vi "Window-Exporting 8bit videos.vi"(9 "Input cluster":T2) -> ()   [LabVIEW 2013]
uses:
  <vilib>/vision/Avi.llb/IMAQ AVI2 Refnum.ctl
  Patch-Vol video generator/Typedefs/Bright-Contr-Gamma cluster.ctl
  Typedefs/Speed graph behaviour enum.ctl
  Typedefs/8-bit video export window ctrl refs.ctl
  Functional Imaging Viewer/Typedefs/Get-Set-Clear Control.ctl
  Patch-Vol video generator/Globals/gl_8-bit montage window ctrl refs.vi
  Globals/gl_Time series viewer globals.vi
  <vilib>/Utility/miscctls.llb/LVPointTypeDef.ctl
panel:
  out "max value":dbl format="Max intensity value: %#_g"
  out "Progress...":u8(slide) scale=0.0..100.0
  out "Progress indicator":string
  out "Pause":bool
  out "Number of frames":i32 format="Number of frames: %.0f"
  out "split file frame index (0 based)":u32
  out "AVI mode":string
  out "Timelapse frame's global number":i32
  out "8-bit":T3(plugin-control) caption="8-bit video to be exported"
  out "16-bit":T3(plugin-control) caption="Original 16-bit video"
  out "AVI2 split file ref":T1
  in  "Include camera videos":bool
  in  "Include speed graph":bool
  in  "Speed graph behaviour":T4
  in  "Micr. Img Adjstmnt":T5={"Brightness"=1000.0, "Contrast"=45.0, "Gamma"=1.0} {"Gamma" min=0.5 scale=0.0..2.0; "Contrast" min=0.5 scale=0.0..90.0; "Brightness" min=0.5 scale=0.0..30000.0}
  out "Stop (ind)":bool
  out "Exporting":bool
  out "Close":bool
  in  "Stop":bool
  in  "Export":bool
  in  "Play":bool
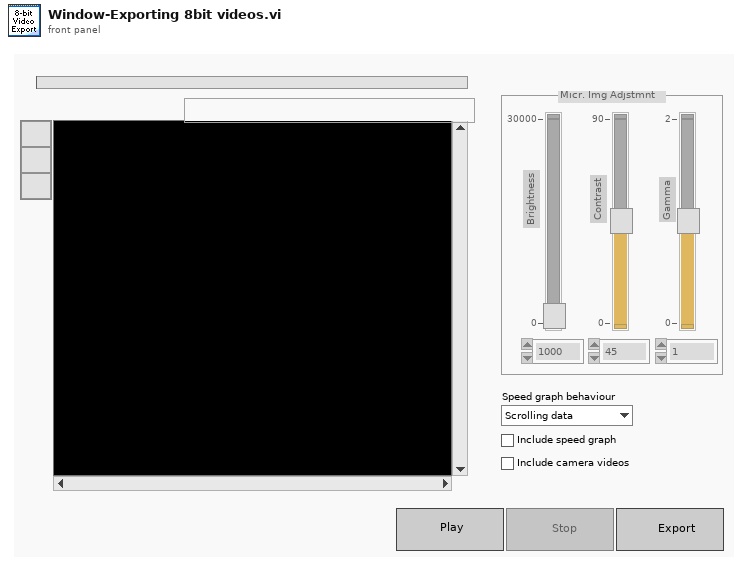
[diagram p1: front panel]
types:
  T1 = typedef "IMAQ AVI2 Refnum.ctl" = refnum<k20>
  T2 = cluster{"# of frames to export":i32, "Initial frame's owning file":T1, "8-bit AVI file path":path, "Cursors location":cluster{"Number of first frame":i32, "Number of last frame":i32}}
  T3 = typedef "IMAQ Image.ctl" = refnum<image>
  T4 = typedef "Speed graph behaviour enum.ctl" = enum16{"Scrolling data", "Scrolling cursor"}
  T5 = typedef "Bright-Contr-Gamma cluster.ctl" = cluster{"Brightness":sgl, "Contrast":sgl, "Gamma":sgl}
  T6 = typedef "8-bit video export window ctrl refs.ctl" = cluster{"Add speed data":refnum<vi>, "Add camera videos":refnum<vi>, "Stop button":refnum<vi>, "Camera Video Adjustments":refnum<vi>, "Microscope Image Adjustments":refnum<vi>, "Execute":refnum<vi>, "Codec":refnum<vi>, "Channel":refnum<vi>, "Speed graph behaviour":refnum<vi>, "Include speed graph":refnum<vi>}
  T7 = cluster{"Number of first frame":i32, "Number of last frame":i32}
  T8 = typedef "LVPointTypeDef.ctl" = cluster{"Horizontal":i16, "Vertical":i16}
  T9 = enum8{"Enabled", "Disabled", "Disabled and Grayed Out"}
  T10 = typedef "Get-Set-Clear Control.ctl" = enum16{"Get", "Set", "Clear"}
  T11 = typedef "Image Type" = u32
  T12 = typedef "AVI modes refs cluster.ctl" = cluster{"AVI1 ref":T13, "AVI2 refs":T1[], "AVI # frames":u32[]}
  T13 = typedef "AviRefnum.ctl" = refnum<k1>
  T14 = enum32{"Invalid", "Standard", "Closed", "Hidden", "Minimized", "Maximized"}
  T15 = typedef "8-bit video export AVI modes cluster.ctl" = cluster{"AVI1 ref":T13, "AVI2 ref":T1, "AVI path":path}
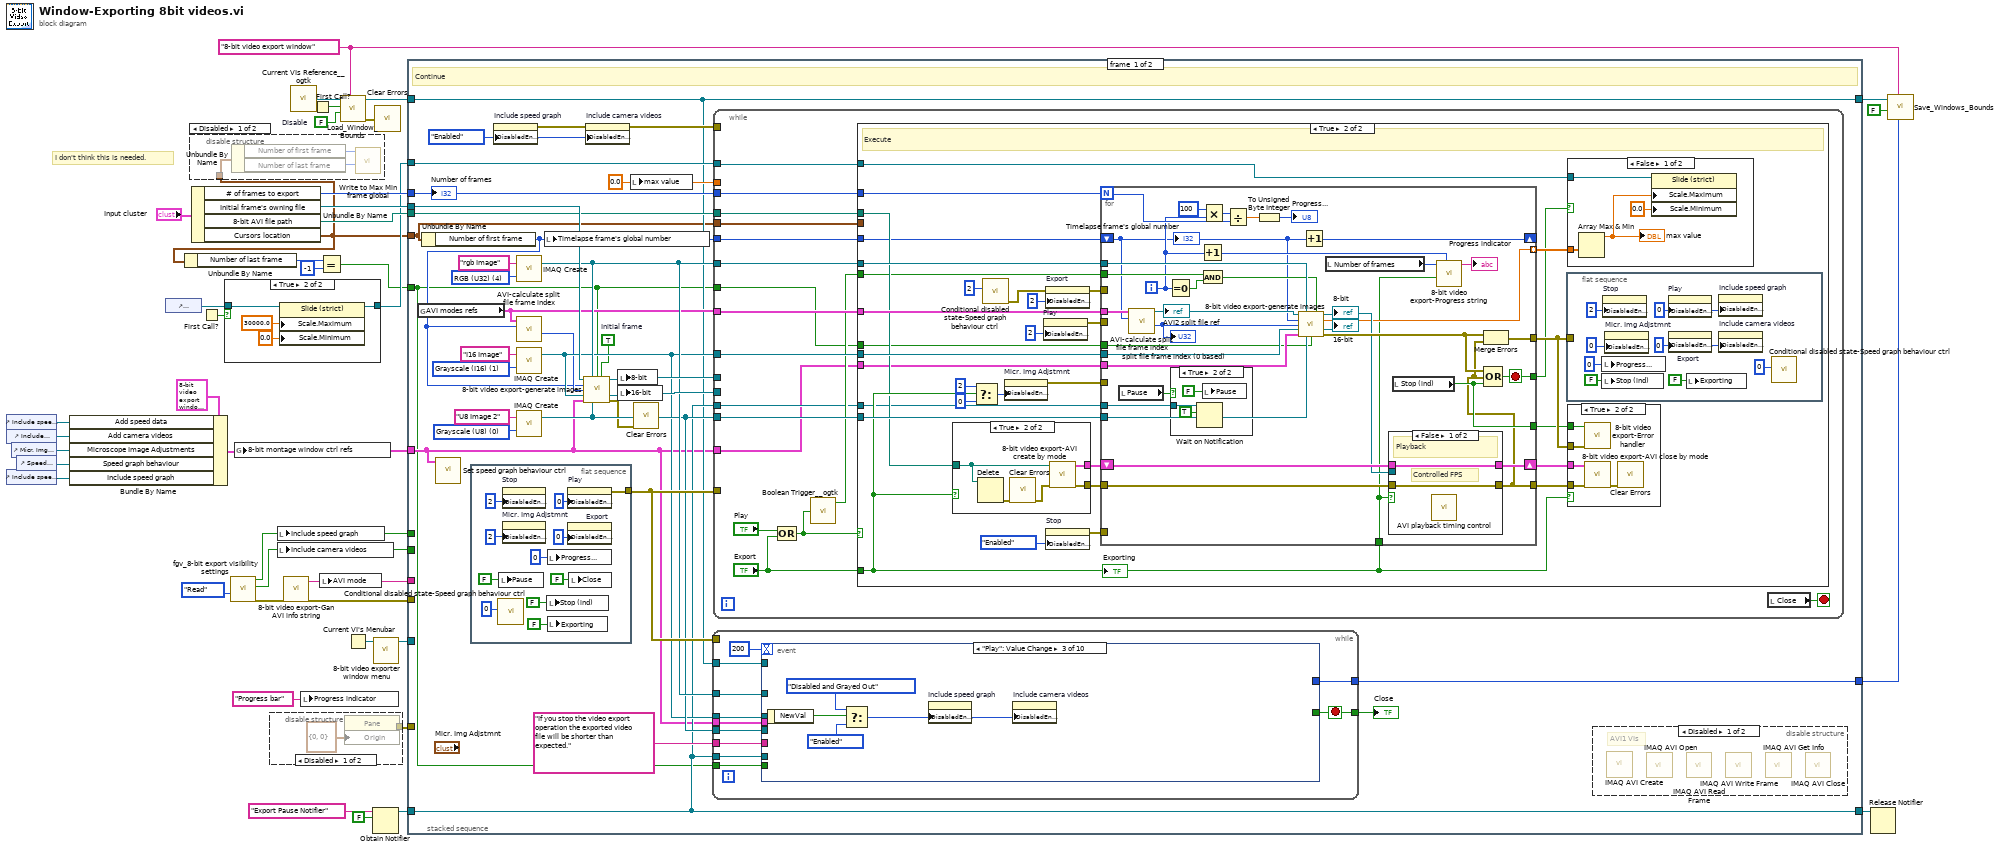
[diagram p0: block diagram]
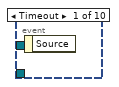
[diagram p6: hidden frame]
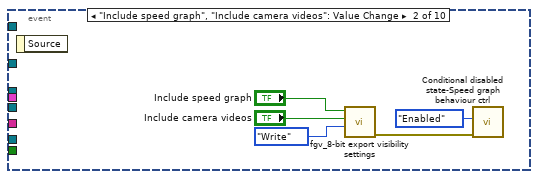
[diagram p7: hidden frame]
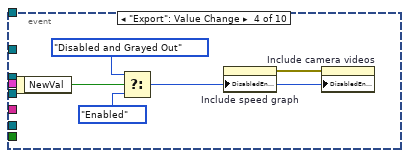
[diagram p8: hidden frame]
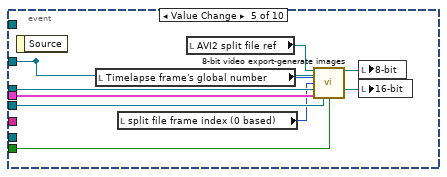
[diagram p9: hidden frame]
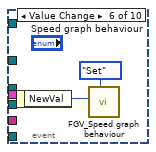
[diagram p10: hidden frame]
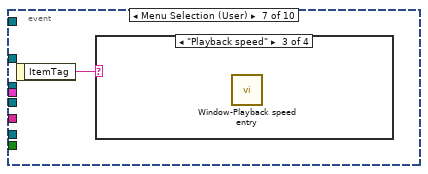
[diagram p11: hidden frame]
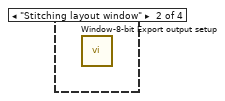
[diagram p13: hidden frame]
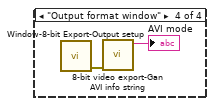
[diagram p14: hidden frame]
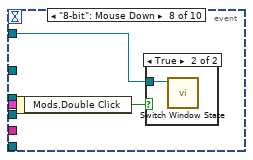
[diagram p15: hidden frame]
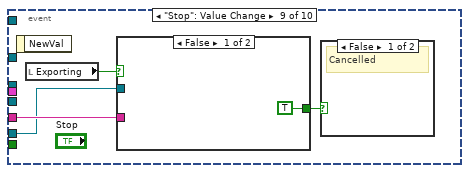
[diagram p17: hidden frame]
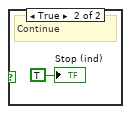
[diagram p18: hidden frame]
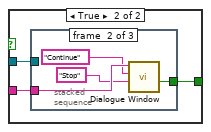
[diagram p19: hidden frame]
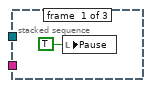
[diagram p20: hidden frame]
diagram:
  w36 = FALSE  # Disable
  w39 = "8-bit video export window" ("Window Name (i.e. Key)")
  # "I don't think this is needed."
  n1 = control-ref of="Include speed graph"() -> (w26:refnum<vi>)
  n2 = control-ref of="Include camera videos"() -> (w25:refnum<vi>)
  n3 = control-ref of="Include speed graph"() -> (w7:refnum<vi>)
  n4 = control-ref of="Micr. Img Adjstmnt"() -> (w12:refnum<vi>)
  n5 = control-ref of="Speed graph behaviour"() -> (w9:refnum<vi>)
  n6 = Bundle By Name(cluster=T6 {"Add speed data"=refnum, "Add camera videos"=refnum, "Stop button"=refnum, "Camera Video Adjustments"=refnum, "Microscope Image Adjustments"=refnum, "Execute"=refnum, "Codec"=refnum, "Channel"=refnum, "Speed graph behaviour"=refnum, "Include speed graph"=refnum} ("output cluster"), "Add speed data"=w26, "Add camera videos"=w25, "Microscope Image Adjustments"=w12, "Speed graph behaviour"=w9, "Include speed graph"=w7) -> (w8:T6)
  n7 = control-ref of="Brightness"() -> (w11:refnum<vi>)
  n8 = Unbundle By Name("Input cluster") -> ("# of frames to export"=w28:i32, "Initial frame's owning file"=w29:T1, "8-bit AVI file path"=w30:path, "Cursors location"=w4:T7)
  n9 = Unbundle By Name(w4) -> ("Number of last frame"=w3:i32)
  n10 = disable-structure shown="Disabled" {
    disable-tunnel: w4 -> [w42 _]
    frame Disabled {
      n11 = Unbundle By Name(w42) -> ("Number of first frame"=w44:i32, "Number of last frame"=w43:i32)
      n12 = call "Write to Max Min frame global.vi"("Max cursor / End frame"=w43, "Min cursor / Start frame"=w44) -> ()  [unwired: 10 in]
    }
    frame Enabled {
    }
  }
  n13 = First Call?() -> (First Call?: T/F=w15:bool)
  n14 = case shown="True" w15 {
    tunnel: w11 -> [w45 w47]
    tunnel: [w45 w46] -> w14
    frame False {
    }
    frame True {
      n15 = property on="Property Node" class="Slide (strict)"(reference=w47, "Scale.Maximum"=30000.0 ("Scale.Range:Maximum"), "Scale.Minimum"=0.0 ("Scale.Range:Minimum")) -> (reference out=w46:refnum<vi>)  [unwired: 1 in, 1 out]
    }
  }
  n16 = call "fgv_8-bit export visibility settings.vi"("Function"=enum16{"Intialize", "Write", "Read", "Clear"}."Read") -> ("error out"=w19:errorcluster, "Include camera videos"=w5:bool, "Include speed graph"=w6:bool)  [unwired: 8 in]
  n17 = global write "gl_8-bit montage window ctrl refs.vi" "8-bit montage window ctrl refs"(w8) -> ()
  n18 = disable-structure shown="Disabled" {
    disable-tunnel: [w50 _] -> w17
    frame Disabled {
      n19 = property class="Pane"("Origin"=T8 {"Horizontal"=0, "Vertical"=0}) -> (reference=w51:refnum<vi>, error out=w50:errorcluster)  [unwired: 1 in, 1 out]
    }
    frame Enabled {
    }
  }
  n20 = local write "Include speed graph"(w6) -> ()
  n21 = local write "Include camera videos"(w5) -> ()
  n22 = call "8-bit video export-Gan AVI info string.vi"("error in (no error)"=w19) -> ("error out"=w21:errorcluster, "Info string"=w18:string)  [unwired: 9 in]
  n23 = call "Current VIs Reference__ogtk.vi"() -> ("Current VI's reference"=w38:refnum<vi>)  [unwired: 5 in]
  n24 = local write "Progress indicator"("Progress bar" ("Progress indicator")) -> ()
  n25 = First Call?() -> (First Call?: T/F=w37:bool)
  n26 = Equal?(x=w3, y=-1) -> (x = y?=w1:bool)
  n27 = local write "AVI mode"(w18) -> ()
  n28 = call "Load_Window_Bounds.vi"("Window Name (i.e. Key)"=w39, "Disable"=w36, "First Call"=w37, "Window VI's Ref"=w38) -> ("error out"=w10:errorcluster, "reference out"=w35:refnum<vi>)  [unwired: 4 in, 2 out]
  n29 = Current VI's Menubar() -> (w23:refnum<k9>)
  n30 = Obtain Notifier(name (unnamed)="Export Pause Notifier", notification data type=FALSE) -> (notifier out=w33:refnum<notifier>)  [unwired: 2 in, 2 out]
  n31 = call "8-bit video exporter window menu.vi"("menu"=w23) -> ("menu reference out"=w22:refnum<k9>)  [unwired: 9 in, 1 out]
  n32 = call <vilib>:"Clear Errors.vi"("error in (no error)"=w10) -> ()  [unwired: 6 in, 1 out]
  n33 = stacked-sequence {
    tunnel: w28 -> [w79 _]
    tunnel: w29 -> [w78 _]
    tunnel: w30 -> [w71 _]
    tunnel: w35 -> [w61 _]
    tunnel: [w61 _] -> w40
    tunnel: w4 -> [w56 _]
    tunnel: [w68 _] -> w34
    tunnel: w33 -> [w68 _]
    tunnel: w8 -> [w55 _]
    tunnel: w22 -> [_ _]
    tunnel: w21 -> [_ _]
    tunnel: w18 -> [_ _]
    tunnel: w17 -> [_ _]
    tunnel: w14 -> [w62 _]
    tunnel: [w60 _] -> w13
    tunnel: w6 -> [_ _]
    tunnel: w5 -> [_ _]
    tunnel: w1 -> [w53 _]
    frame #0 {
      w54 = TRUE  # Initial frame
      w66 = T9."Enabled" ("Disabled")
      w80 = 0.0 ("max value")
      w57 = T11 0 items=["Grayscale (U8)", "Grayscale (I16)", "Grayscale (SGL)", "Complex (CSG)", "RGB (U32)", "HSL (U32)", "RGB (U64)", "Grayscale (U16)"] ("Image Type")
      w82 = T11 1 items=["Grayscale (U8)", "Grayscale (I16)", "Grayscale (SGL)", "Complex (CSG)", "RGB (U32)", "HSL (U32)", "RGB (U64)", "Grayscale (U16)"] ("Image Type")
      w85 = T11 4 items=["Grayscale (U8)", "Grayscale (I16)", "Grayscale (SGL)", "Complex (CSG)", "RGB (U32)", "HSL (U32)", "RGB (U64)", "Grayscale (U16)"] ("Image Type")
      # "Continue"
      n34 = global read "gl_Time series viewer globals.vi" "AVI modes refs"() -> (w63:T12)
      n35 = Unbundle By Name(w56) -> ("Number of first frame"=w58:i32)
      n36 = call "Set speed graph behaviour ctrl.vi"("Exporter's ctrl refs"=w55) -> ()  [unwired: 10 in, 1 out]
      n37 = flat-sequence {
        tunnel: [w173] -> w75
        frame #0 {
          n38 = call "Conditional disabled state-Speed graph behaviour ctrl.vi"("Disabled"=0) -> ()  [unwired: 10 in, 1 out]
          n39 = local write "Pause"(FALSE ("Pause")) -> ()
          n40 = property on="Stop" class="Bool"("DisabledEnum"=2) -> ()  [unwired: 2 in, 2 out]
          n41 = property on="Micr. Img Adjstmnt" class="Clust (strict)"("DisabledEnum"=2) -> ()  [unwired: 2 in, 2 out]
          n42 = local write "Stop (ind)"(FALSE ("Stop (ind)")) -> ()
          n43 = local write "Progress..."(u8 0 ("Progress...")) -> ()
          n44 = local write "Exporting"(FALSE ("Exporting")) -> ()
          n45 = property on="Play" class="Bool"("DisabledEnum"=0) -> (error out=w173:errorcluster)  [unwired: 2 in, 1 out]
          n46 = property on="Export" class="Bool"("DisabledEnum"=0) -> ()  [unwired: 2 in, 2 out]
          n47 = local write "Close"(FALSE ("Stop")) -> ()
        }
      }
      n48 = property on="Include speed graph" class="Bool (strict)"("DisabledEnum"=w66) -> (error out=w65:errorcluster)  [unwired: 2 in, 1 out]
      n49 = call "IMAQ Create"("Image Name"="rgb Image", "Image Type"=w85) -> ("New Image"=w72:T3)  [unwired: 2 in, 2 out]
      n50 = call "AVI-calculate split file frame index.vi"("Frame number (unity-based) in"=w58, "AVI modes refs"=w63) -> ("Index of frame in split file"=w59:u32)  [unwired: 6 in, 3 out]
      n51 = call "IMAQ Create"("Image Name"="I16 Image", "Image Type"=w82) -> ("New Image"=w69:T3)  [unwired: 2 in, 2 out]
      n52 = call "IMAQ Create"("Image Name"="U8 Image 2", "Image Type"=w57) -> ("New Image"=w70:T3)  [unwired: 2 in, 2 out]
      n53 = local write "Timelapse frame's global number"(w58) -> ()
      n54 = call "8-bit video export-generate images.vi"("AVI2 split file ref"=w78, "rgb Image"=w72, "Initial frame"=w54, "Gobal frame number in time series data /master video (1 based)"=w58, "Split time series file frame index (0 based)"=w59, "I16 Image ref in"=w69, "Ctrl refs"=w55, "U8 Image ref in"=w70, "Whole dataset"=w53) -> ("U8 Image"=w77:T3, "I16 Image"=w76:T3, "error out"=w67:errorcluster)  [unwired: 3 in, 1 out]
      n55 = property on="Include camera videos" class="Bool (strict)"(error in=w65, "DisabledEnum"=w66) -> (error out=w64:errorcluster)  [unwired: 1 in, 1 out]
      n56 = local write "8-bit"(w77) -> ()
      n57 = local write "16-bit"(w76) -> ()
      n58 = local write "max value"(w80) -> ()
      n59 = call <vilib>:"Clear Errors.vi"("error in (no error)"=w67) -> ()  [unwired: 6 in, 1 out]
      n60 = while {
        tunnel: w75 -> [_]
        tunnel: [w95] -> w74
        tunnel: "If you stop the video export operation the exported video file will be shorter than expected." ("Message string") -> [w94]
        tunnel: w72 -> [w93]
        tunnel: w70 -> [w92]
        tunnel: w69 -> [w91]
        tunnel: w68 -> [w90]
        tunnel: w55 -> [w89]
        tunnel: w61 -> [w88]
        tunnel: [w87] -> w60
        tunnel: w53 -> [w86]
        stop <- w95 stop-if-true
        n61 = event shown="[2] \"Play\": Value Change" {
          selector: _ -> [_ _ _ _ _ _ _ _ _ _]
          dyn-events: _ -> [_ _ _ _ _ _ _ _ _ _]
          timeout: 200 -> [_ _ _ _ _ _ _ _ _ _]
          tunnel: [_ _ _ _ _ _ _ _ _ w152] -> w95
          tunnel: w94 -> [_ _ _ _ _ _ _ _ w131 w149]
          tunnel: [_ _ _ _ w118 _ _ _ _ _] -> _
          tunnel: w93 -> [_ _ _ _ w118 _ _ _ _ _]
          tunnel: w92 -> [_ _ _ _ w116 _ _ _ _ _]
          tunnel: w91 -> [_ _ _ _ w115 _ _ _ _ _]
          tunnel: w90 -> [_ _ _ _ _ _ _ _ w129 w148]
          tunnel: w89 -> [_ _ _ _ w114 _ _ _ _ _]
          tunnel: w88 -> [_ _ _ _ _ _ _ w126 _ w147]
          tunnel: [_ _ _ _ _ _ _ _ _ w146] -> w87
          tunnel: w86 -> [_ _ _ _ w111 _ _ _ _ _]
          event Timeout {
            n62 = event-data() -> ()  [unwired: 1 in, 1 out]
          }
          event "Include speed graph", "Include camera videos": Value Change {
            n63 = event-data() -> ()  [unwired: 1 in, 1 out]
            n64 = call "fgv_8-bit export visibility settings.vi"("Function"=enum16{"Intialize", "Write", "Read", "Clear"}."Write", "Include camera videos"="Include camera videos", "Include speed graph"="Include speed graph") -> ("error out"=w98:errorcluster)  [unwired: 6 in, 2 out]
            n65 = call "Conditional disabled state-Speed graph behaviour ctrl.vi"("error in (no error)"=w98, "Disabled"=T9."Enabled") -> ()  [unwired: 9 in, 1 out]
          }
          event "Play": Value Change {
            n66 = event-data() -> ("NewVal"=w105:bool)  [unwired: 1 in]
            n67 = Select(t=T9."Disabled and Grayed Out" ("Disabled"), s=w105, f=T9."Enabled" ("Disabled")) -> (s? t:f=w102:T9)
            n68 = property on="Include speed graph" class="Bool (strict)"("DisabledEnum"=w102) -> ()  [unwired: 2 in, 2 out]
            n69 = property on="Include camera videos" class="Bool (strict)"("DisabledEnum"=w102) -> ()  [unwired: 2 in, 2 out]
          }
          event "Export": Value Change {
            n70 = event-data() -> ("NewVal"=w108:bool)  [unwired: 1 in]
            n71 = Select(t=T9."Disabled and Grayed Out" ("Disabled"), s=w108, f=T9."Enabled" ("Disabled")) -> (s? t:f=w107:T9)
            n72 = property on="Include speed graph" class="Bool (strict)"("DisabledEnum"=w107) -> (error out=w106:errorcluster)  [unwired: 2 in, 1 out]
            n73 = property on="Include camera videos" class="Bool (strict)"(error in=w106, "DisabledEnum"=w107) -> ()  [unwired: 1 in, 2 out]
          }
          event Value Change {
            n74 = event-data() -> ()  [unwired: 1 in, 1 out]
            n75 = local read "Timelapse frame's global number"() -> (w112:i32)
            n76 = local read "split file frame index (0 based)"() -> (w113:u32)
            n77 = local read "AVI2 split file ref"() -> (w117:T1)
            n78 = call "8-bit video export-generate images.vi"("AVI2 split file ref"=w117, "rgb Image"=w118, "Gobal frame number in time series data /master video (1 based)"=w112, "Split time series file frame index (0 based)"=w113, "I16 Image ref in"=w115, "Ctrl refs"=w114, "U8 Image ref in"=w116, "Whole dataset"=w111) -> ("U8 Image"=w119:T3, "I16 Image"=w120:T3)  [unwired: 4 in, 2 out]
            n79 = local write "8-bit"(w119) -> ()
            n80 = local write "16-bit"(w120) -> ()
          }
          event Value Change {
            n81 = event-data() -> ("NewVal"=w121:T4)  [unwired: 1 in]
            n82 = call "FGV_Speed graph behaviour.vi"("Function"=Get-Set-Clear_Control."Set", "Speed graph behaviour"=w121) -> ()  [unwired: 8 in, 2 out]
          }
          event Menu Selection (User) {
            n83 = event-data() -> ("ItemTag"=w123:string)  [unwired: 1 in]
            n84 = case shown="\"Playback speed\"" w123 {
              frame Default {
              }
              frame "Stitching layout window" {
                n85 = call "Window-8-bit Export output setup.vi"() -> ()  [unwired: 12 in]
              }
              frame "Playback speed" {
                n86 = call "Window-Playback speed entry.vi"() -> ()  [unwired: 10 in, 2 out]
              }
              frame "Output format window" {
                n87 = call "Window-8-bit Export-Output setup.vi"() -> ("error out (no error)"=w124:errorcluster)  [unwired: 11 in]
                n88 = call "8-bit video export-Gan AVI info string.vi"("error in (no error)"=w124) -> ("Info string"=→"AVI mode":string)  [unwired: 9 in, 1 out]
              }
            }
          }
          event "8-bit": Mouse Down {
            n89 = event-data() -> ("Mods.Double Click"=w127:bool)  [unwired: 1 in]
            n90 = case shown="True" w127 {
              tunnel: w126 -> [_ w128]
              frame False {
              }
              frame True {
                n91 = call "Switch Window State.vi"("Window VI's Ref"=w128) -> ()  [unwired: 10 in, 1 out]
              }
            }
          }
          event "Stop": Value Change {
            n92 = event-data() -> ()  [unwired: 1 in, 1 out]
            n93 = local read "Exporting"() -> (w132:bool)
            n94 = case shown="False" w132 {
              tunnel: [TRUE ("Cancelled (Left button pressed)") w137] -> w130
              tunnel: w131 -> [_ w136]
              tunnel: w129 -> [_ w135]
              frame False {
              }
              frame True {
                n95 = stacked-sequence {
                  tunnel: [_ w142 _] -> w137
                  tunnel: w136 -> [_ w141 _]
                  tunnel: w135 -> [_ _ w144]
                  frame #0 {
                    n96 = local write "Pause"(TRUE ("Pause")) -> ()
                  }
                  frame #1 {
                    n97 = call "Dialogue Window.vi"("Caption-Left button (Cancel)"="Stop", "Caption-Right button (OK)"="Continue", "Message string"=w141) -> ("Cancelled (Left button pressed)"=w142:bool)  [unwired: 6 in, 2 out]
                  }
                  frame #2 {
                    n98 = Send Notification(notification=FALSE, notifier=w144) -> ()  [unwired: 1 in, 2 out]
                  }
                }
              }
            }
            n99 = case shown="False" w130 {
              frame False {
                # "Cancelled"
              }
              frame True {
                # "Continue"
                "Stop (ind)" <- TRUE ("Stop (ind)")
              }
            }
          }
          event Panel Close? {
            n100 = event-data() -> ()  [unwired: 1 in, 1 out]
            n101 = local read "Exporting"() -> (w150:bool)
            n102 = case shown="True" w150 {
              tunnel: [TRUE ("Cancelled (Left button pressed)") w156] -> w151
              tunnel: w149 -> [_ w155]
              tunnel: w148 -> [_ w154]
              frame False {
              }
              frame True {
                n103 = stacked-sequence {
                  tunnel: [_ w159 _] -> w156
                  tunnel: w155 -> [_ w158 _]
                  tunnel: w154 -> [_ _ w163]
                  frame #0 {
                    "Pause" <- TRUE ("Pause")
                  }
                  frame #1 {
                    n104 = call "Dialogue Window.vi"("Caption-Left button (Cancel)"="Close", "Caption-Right button (OK)"="Continue", "Message string"=w158) -> ("Cancelled (Left button pressed)"=w159:bool)  [unwired: 6 in, 2 out]
                  }
                  frame #2 {
                    n105 = Send Notification(notification=FALSE, notifier=w163) -> ()  [unwired: 1 in, 2 out]
                  }
                }
              }
            }
            n106 = case shown="True" w151 {
              tunnel: [FALSE w165] -> w152
              frame False {
                # "Cancelled"
              }
              frame True {
                w165 = TRUE
                # "Stop & close window"
                n107 = local write "Stop (ind)"(w165) -> ()
              }
            }
            n108 = property class="VI"(reference=w147) -> ("FP.State"=w146:T14)  [unwired: 1 in, 2 out]
            n109 = event-data("Discard?"=TRUE) -> ()  [unwired: 1 in, 1 out]
          }
        }
      }
      "Close" <- w74
      n110 = while {
        tunnel: w72 -> [w193]
        tunnel: w69 -> [w192]
        tunnel: w70 -> [w191]
        tunnel: w80 -> [_]
        tunnel: w79 -> [w190]
        tunnel: w63 -> [w189]
        tunnel: w77 -> [_]
        tunnel: w76 -> [_]
        tunnel: w75 -> [_]
        tunnel: w71 -> [w186]
        tunnel: w58 -> [w182]
        tunnel: w62 -> [w181]
        tunnel: w68 -> [w180]
        tunnel: w55 -> [w179]
        tunnel: w64 -> [_]
        tunnel: w56 -> [w178]
        tunnel: w53 -> [w177]
        stop <- w187 stop-if-true
        n111 = Compound Arithmetic op=OR("Play", "Export") -> (w184:bool)
        n112 = call "Boolean Trigger__ogtk.vi"("Boolean Input"=w184) -> ("Rising Edge"=w183:bool)  [unwired: 1 in, 1 out]
        n113 = case shown="True" w184 {
          tunnel: w193 -> [w200 w247]
          tunnel: w192 -> [w199 w246]
          tunnel: w191 -> [w198 w245]
          tunnel: w186 -> [_ w231]
          tunnel: "Export" -> [_ w234]
          tunnel: w190 -> [_ w226]
          tunnel: w189 -> [w201 w242]
          tunnel: w183 -> [_ w227]
          tunnel: w182 -> [_ w221]
          tunnel: w181 -> [_ w225]
          tunnel: w180 -> [_ w223]
          tunnel: w179 -> [w197 w218]
          tunnel: w178 -> [_ _]
          tunnel: w177 -> [w194 w215]
          frame False {
            # "Idle"
            n114 = global read "gl_Time series viewer globals.vi" "Layout change"() -> (w195:bool)
            n115 = case shown="True" w195 {
              tunnel: w201 -> [_ w209]
              tunnel: w200 -> [_ w207]
              tunnel: w199 -> [_ w206]
              tunnel: w198 -> [_ w205]
              tunnel: w197 -> [_ w204]
              tunnel: w194 -> [_ w202]
              frame False {
              }
              frame True {
                # "This case refreshes the image to make it update while the user plays around with the layout setup."
                # "The Layout setup window is open."
                n116 = local read "Timelapse frame's global number"() -> (w211:i32)
                n117 = call "AVI-calculate split file frame index.vi"("Frame number (unity-based) in"=w211, "AVI modes refs"=w209) -> ("Index of frame in split file"=w213:u32, "index of  split file"=w212:i32, "AVI2 split file ref"=w208:T1)  [unwired: 6 in, 1 out]
                n118 = call "8-bit video export-generate images.vi"("AVI2 split file ref"=w208, "rgb Image"=w207, "Initial frame"=TRUE, "Gobal frame number in time series data /master video (1 based)"=w212, "Split time series file frame index (0 based)"=w213, "I16 Image ref in"=w206, "Ctrl refs"=w204, "U8 Image ref in"=w205, "Whole dataset"=w202) -> ("U8 Image"=w210:T3)  [unwired: 3 in, 3 out]
                n119 = global write "gl_Time series viewer globals.vi" "Layout change"(FALSE ("Layout change")) -> ()
                n120 = local write "8-bit"(w210) -> ()
              }
            }
            n121 = Wait Until Next ms Multiple(millisecond multiple=u32 200) -> ()  [unwired: 1 out]
          }
          frame True {
            # "Execute"
            n122 = case shown="True" w234 {
              tunnel: [_ w313] -> w243
              tunnel: [_ w312] -> w230
              tunnel: w231 -> [_ w314]
              frame False {
              }
              frame True {
                n123 = Delete(path (use dialog)=w314) -> (error out=w315:errorcluster)  [unwired: 4 in, 2 out]
                n124 = call <vilib>:"Clear Errors.vi"("error in (no error)"=w315) -> ("error out"=w311:errorcluster)  [unwired: 6 in]
                n125 = call "8-bit video export-AVI create by mode.vi"("error in (no error)"=w311, "8-bit AVI file path"=w314) -> ("error out"=w312:errorcluster, "AVI modes refs"=w313:T15)  [unwired: 8 in]
              }
            }
            n126 = Select(t=2, s=w234, f=0) -> (s? t:f=w220:i32)
            n127 = call "Conditional disabled state-Speed graph behaviour ctrl.vi"("Disabled"=2) -> ("error out"=w217:errorcluster)  [unwired: 10 in]
            n128 = property on="Micr. Img Adjstmnt" class="Clust (strict)"("DisabledEnum"=w220) -> (error out=w219:errorcluster)  [unwired: 2 in, 1 out]
            n129 = property on="Play" class="Bool"("DisabledEnum"=2) -> (error out=w235:errorcluster)  [unwired: 2 in, 1 out]
            n130 = property on="Export" class="Bool"(error in=w217, "DisabledEnum"=2) -> (error out=w236:errorcluster)  [unwired: 1 in, 1 out]
            n131 = property on="Stop" class="Bool"("DisabledEnum"=T9."Enabled" ("Disabled")) -> (error out=w240:errorcluster)  [unwired: 2 in, 1 out]
            n132 = for {
              N: w226 -> [w273]
              tunnel: w247 -> [w280]
              tunnel: w246 -> [w287]
              tunnel: w245 -> [w279]
              shift-right: [w286] -> w244
              shift-left: w243 -> [w285]
              tunnel: [w276] -> w241 mode=indexing
              tunnel: w234 -> [w259]
              tunnel: [w283] -> w228
              tunnel: w242 -> [w282]
              tunnel: [w281] -> w224
              tunnel: w240 -> [_]
              tunnel: w236 -> [_]
              tunnel: w235 -> [_]
              tunnel: w230 -> [w270]
              tunnel: [w253] -> w229
              tunnel: w218 -> [w263]
              tunnel: w227 -> [w269]
              shift-right: [w256] -> _
              shift-left: w221 -> [w254]
              tunnel: w223 -> [w265]
              tunnel: [w264] -> w222
              tunnel: w219 -> [_]
              tunnel: w215 -> [w252]
              i -> [w258]
              stop <- w281 stop-if-true
              n133 = local read "Pause"() -> (w266:bool)
              n134 = call "AVI-calculate split file frame index.vi"("Frame number (unity-based) in"=w254, "AVI modes refs"=w282) -> ("Index of frame in split file"=w255:u32, "AVI2 split file ref"=w262:T1)  [unwired: 6 in, 2 out]
              "split file frame index (0 based)" <- w255
              "AVI2 split file ref" <- w262
              n135 = Equal To 0?(x=w258) -> (x = 0?=w267:bool)
              n136 = case shown="True" w266 {
                tunnel: w265 -> [_ w290]
                frame False {
                }
                frame True {
                  n137 = Wait on Notification(notifier=w290, ignore previous (F)=TRUE) -> ()  [unwired: 2 in, 4 out]
                  n138 = local write "Pause"(FALSE ("Pause")) -> ()
                }
              }
              n139 = Increment(x=w258) -> (x+1=w257:i32)
              n140 = And(x=w269, y=w267) -> (x .and. y?=w268:bool)
              n141 = Multiply(x=100, y=w258) -> (x*y=w274:i32)
              n142 = Divide(x=w274, y=w273) -> (x/y=w272:dbl)
              n143 = To Unsigned Byte Integer(number=w272) -> (unsigned 8bit integer=→"Progress...":u8)
              n144 = call "8-bit video export-generate images.vi"("AVI2 split file ref"=w262, "rgb Image"=w280, "Initial frame"=w268, "Gobal frame number in time series data /master video (1 based)"=w254, "Split time series file frame index (0 based)"=w255, "I16 Image ref in"=w287, "Ctrl refs"=w263, "U8 Image ref in"=w279, "Whole dataset"=w252) -> ("U8 Image"=w277:T3, "Max intensity value"=w276:dbl, "I16 Image"=→"16-bit":T3, "error out"=w284:errorcluster)  [unwired: 3 in]
              "8-bit" <- w277
              n145 = Increment(x=w254) -> (x+1=w256:i32)
              n146 = local read "Number of frames"() -> (w261:i32)
              n147 = case shown="False" w259 {
                tunnel: [w292 w296] -> w286
                tunnel: w285 -> [w292 w293]
                tunnel: w270 -> [w291 w297]
                tunnel: [w291 w295] -> w253
                tunnel: w277 -> [_ w294]
                frame False {
                  # "Controlled FPS"
                  # "Playback"
                  n148 = call "AVI playback timing control.vi"() -> ()  [unwired: 8 in, 4 out]
                }
                frame True {
                  # "as fast as possible"
                  # "Exporting"
                  n149 = call "8-bit video export-AVI write by mode.vi"("error in (no error)"=w297, "RGB image ref in"=w294, "AVI modes refs"=w293) -> ("error out"=w295:errorcluster, "AVI modes refs"=w296:T15)  [unwired: 7 in]
                }
              }
              n150 = local read "Stop (ind)"() -> (w264:bool)
              n151 = call "8-bit video export-Progress string.vi"("Currnet frame number in selected chunk (1based)"=w257, "Exporting"=w259, "Number of frames in selected chunk"=w261) -> ("Progress string"=→"Progress indicator":string)  [unwired: 8 in]
              n152 = Merge Errors(w284, w253) -> (w283:errorcluster)
              n153 = Compound Arithmetic op=OR(w284, w253, w264) -> (w281:bool)
              "Timelapse frame's global number" <- w254
            }
            n154 = flat-sequence {
              tunnel: w228 -> [_]
              frame #0 {
                w300 = 0
                w301 = 0
                n155 = local write "Progress..."(u8 0 ("Progress...")) -> ()
                n156 = local write "Stop (ind)"(FALSE ("Stop (ind)")) -> ()
                n157 = property on="Stop" class="Bool"("DisabledEnum"=2) -> ()  [unwired: 2 in, 2 out]
                n158 = property on="Micr. Img Adjstmnt" class="Clust (strict)"("DisabledEnum"=0) -> ()  [unwired: 2 in, 2 out]
                n159 = property on="Play" class="Bool"("DisabledEnum"=w301) -> ()  [unwired: 2 in, 2 out]
                n160 = property on="Export" class="Bool"("DisabledEnum"=w300) -> ()  [unwired: 2 in, 2 out]
                n161 = local write "Exporting"(FALSE ("Exporting")) -> ()
                n162 = property on="Include speed graph" class="Bool (strict)"("DisabledEnum"=w301) -> ()  [unwired: 2 in, 2 out]
                n163 = property on="Include camera videos" class="Bool (strict)"("DisabledEnum"=w300) -> ()  [unwired: 2 in, 2 out]
                n164 = call "Conditional disabled state-Speed graph behaviour ctrl.vi"("Disabled"=0) -> ()  [unwired: 10 in, 1 out]
              }
            }
            n165 = case shown="False" w224 {
              tunnel: w241 -> [w251 _]
              tunnel: w225 -> [w248 _]
              frame False {
                n166 = Array Max & Min(array=w251) -> (max value=w250:dbl)  [unwired: 3 out]
                "max value" <- w250
                n167 = property on="Property Node" class="Slide (strict)"(reference=w248, "Scale.Maximum"=w250, "Scale.Minimum"=0.0 ("Scale.Range:Minimum")) -> ()  [unwired: 1 in, 2 out]
              }
              frame True {
              }
            }
            n168 = case shown="True" w234 {
              tunnel: w244 -> [_ w308]
              tunnel: w229 -> [_ w307]
              tunnel: w228 -> [_ w310]
              tunnel: w222 -> [_ w309]
              frame False {
              }
              frame True {
                n169 = call "8-bit video export-Error handler.vi"("error in (no error)"=w310, "Stop"=w309) -> ()  [unwired: 10 in]
                n170 = call "8-bit video export-AVI close by mode.vi"("error in (no error)"=w307, "AVI modes refs"=w308) -> ("error out"=w306:errorcluster)  [unwired: 8 in, 1 out]
                n171 = call <vilib>:"Clear Errors.vi"("error in (no error)"=w306) -> ()  [unwired: 6 in, 1 out]
              }
            }
            "Exporting" <- w234
          }
        }
        n172 = local read "Close"() -> (w187:bool)
      }
      n173 = disable-structure shown="Disabled" {
        frame Disabled {
          # "AVI1 VIs"
          n174 = call "IMAQ AVI Create"() -> ()  [unwired: 10 in, 2 out]
          n175 = call "IMAQ AVI Open"() -> ()  [unwired: 10 in, 2 out]
          n176 = call "IMAQ AVI Read Frame"() -> ()  [unwired: 8 in, 4 out]
          n177 = call "IMAQ AVI Write Frame"() -> ()  [unwired: 10 in, 2 out]
          n178 = call "IMAQ AVI Get Info"() -> ()  [unwired: 7 in, 5 out]
          n179 = call "IMAQ AVI Close"() -> ()  [unwired: 11 in, 1 out]
        }
        frame Enabled {
        }
      }
      "Number of frames" <- w79
    }
    frame #1 {
      # "Cancelled"
    }
  }
  n180 = Release Notifier(notifier=w34) -> ()  [unwired: 2 in, 3 out]
  n181 = call "Save_Windows_Bounds.vi"("FP.State"=w13, "Window Name (i.e. Key)"=w39, "Front Panel Window:Open"=FALSE, "Window VI's Ref"=w40) -> ()  [unwired: 7 in, 1 out]
